vi "Teleop.vi"(10 "Match Info":T1={"Autonomous Elapsed Seconds"=0.0, "TeleOp Elapsed Seconds"=0.0, "Disabled Elapsed Seconds"=0.0, "Visited Autonomous"=FALSE, "Visited TeleOp"=FALSE, "Visited Disabled"=FALSE, "Autonomous Settings"={"Autonomous Style"=enum."Independent", "VI Refnum"=refnum}}, 11 "Call Context":T2) -> ()   [LabVIEW 2013]
doc: "This VI is called for each TeleOp packet received from the DS where the robot is not disabled. It is often used to read from the joysticks and update I/O or to update setpoints for timed control loops. It should complete and return within 20 milliseconds or it may miss DS packets."
uses:
  <vilib>/Rock Robotics/WPI/DriverStation/WPI_DriverStationDerivedRobotMode.ctl
  <vilib>/Rock Robotics/WPI/DriverStation/WPI_DriverStationMatch Info.ctl
  <vilib>/Rock Robotics/WPI/Relay/WPI_RelayValue.ctl
  <vilib>/Rock Robotics/WPI/DriverStation/DriverStationLCD/WPI_DriverStationLCDLCDLine.ctl
  <vilib>/Rock Robotics/WPI/Solenoid/WPI_SolenoidValue.ctl
  Robot Global Data.vi
  <vilib>/Rock Robotics/WPI/Solenoid/WPI_SolenoidSetEnum.vi
  <vilib>/Rock Robotics/WPI/Joystick/WPI_JoystickGetSetRefNum.vi
  <vilib>/Rock Robotics/WPI/Compressor/WPI_CompressorGetSetRefNum.vi
  <vilib>/Rock Robotics/WPI/RobotDrive/WPI_RobotDriveGetSetRefNum.vi
panel:
  out "Numeric 1":dbl(slide) scale=0.0..100.0
  out "Boolean 2":bool
  out "Boolean 1":bool
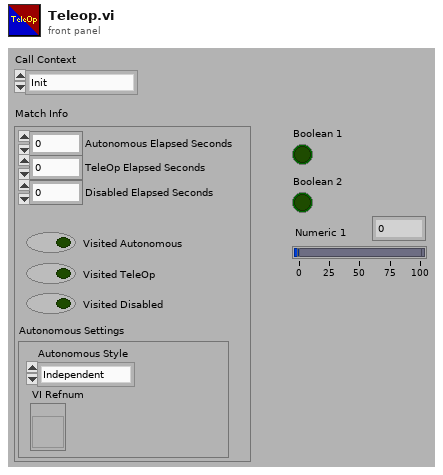
[diagram p1: front panel]
types:
  T1 = typedef "WPI_DriverStationMatch Info.ctl" = cluster{"Autonomous Elapsed Seconds":dbl, "TeleOp Elapsed Seconds":dbl, "Disabled Elapsed Seconds":dbl, "Visited Autonomous":bool, "Visited TeleOp":bool, "Visited Disabled":bool, "Autonomous Settings":cluster{"Autonomous Style":enum16{"Iterative", "Independent"}, "VI Refnum":refnum<vi>}}
  T2 = typedef "WPI_DriverStationDerivedRobotMode.ctl" = enum16{"Init", "Execute", "Stop"}
  T3 = typedef "WPI_JoystickDevRef.ctl" = cluster{"Device":T4}
  T4 = typedef "WPI_JoystickDeviceEnum.ctl" = enum16{"USB 1", "USB 2", "USB 3", "USB 4", "Kinect 1", "Kinect 2"}
  T5 = typedef "WPI_JoystickButtonState.ctl" = cluster{"Button 1":bool, "Button 2":bool, "Button 3":bool, "Button 4":bool, "Button 5":bool, "Button 6":bool, "Button 7":bool, "Button 8":bool, "Button 9":bool, "Button 10":bool, "Button 11":bool, "Button 12":bool}
  T6 = cluster{"axis 1 (x)":dbl, "axis 2 (y)":dbl, "axis 3 (throttle)":dbl, "axis 4":dbl, "axis 5":dbl, "axis 6":dbl}
  T7 = cluster{"Driver Station Digital Input (1-8)[0]":bool, "Driver Station Digital Input (1-8)[1]":bool, "Driver Station Digital Input (1-8)[2]":bool, "Driver Station Digital Input (1-8)[3]":bool, "Driver Station Digital Input (1-8)[4]":bool, "Driver Station Digital Input (1-8)[5]":bool, "Driver Station Digital Input (1-8)[6]":bool, "Driver Station Digital Input (1-8)[7]":bool, "Driver Station Digital Input (1-8)[8]":bool}
  T8 = typedef "WPI_CompressorDevRef.ctl" = cluster{"DevStatus":errorcluster, "DigitalInputDevRef":T9, "RelayDevRef":T12}
  T9 = typedef "WPI_DigitalInputDevRef.ctl" = cluster{"DevStatus":errorcluster, "DIO Channel":T10, "Digital Module":T11}
  T10 = typedef "FPGA_DIOChannel.ctl" = enum8{"DIO 1", "DIO 2", "DIO 3", "DIO 4", "DIO 5", "DIO 6", "DIO 7", "DIO 8", "DIO 9", "DIO 10", "DIO 11", "DIO 12", "DIO 13", "DIO 14", "Invalid"}
  T11 = typedef "FPGA_TypedefDigitalModule.ctl" = enum16{"Digital Module 1", "Digital Module 2"}
  T12 = typedef "WPI_RelayDevRef.ctl" = cluster{"DevStatus":errorcluster, "Relay Channel":T13, "Digital Module":T11, "Relay Direction":T14}
  T13 = typedef "FPGA_DIORelayChannel.ctl" = enum8{"Relay 1", "Relay 2", "Relay 3", "Relay 4", "Relay 5", "Relay 6", "Relay 7", "Relay 8", "Invalid"}
  T14 = typedef "WPI_RelayDirection.ctl" = enum16{"Both directions", "Forward only", "Reverse only"}
  T15 = typedef "WPI_SolenoidValue.ctl" = enum16{"Off", "On", "Forward", "Reverse"}
  T16 = typedef "WPI_DriverStationLCDLCDLine.ctl" = enum16{"Main - Line 1", "User - Line 2", "User - Line 3", "User - Line 4", "User - Line 5", "User - Line 6"}
  T17 = typedef "WPI_RelayValue.ctl" = enum16{"Off", "On", "Forward", "Reverse"}
  T18 = typedef "WPI_RobotDriveDevRef.ctl" = cluster{"DevStatus":errorcluster, "Motors[]":T19[], "Square Inputs":bool, "Max Output":dbl, "Isochronous":bool}
  T19 = typedef "WPI_MotorControlDeviceRef.ctl" = cluster{"DeviceStatus":errorcluster, "Type":enum16{"PWM", "CAN"}, "PWM":cluster{"Digital Module":T11, "PWM Channel":T20, "DeadBand":T21}, "CAN":cluster{"Device Number":u8, "Control Mode":T22, "Semaphore":T23, "Max Vout":dbl}, "Invert":bool, "TransformRef":T24, "InvTransformRef":T24}
  T20 = typedef "FPGA_DIOPWMChannel.ctl" = enum8{"PWM 1", "PWM 2", "PWM 3", "PWM 4", "PWM 5", "PWM 6", "PWM 7", "PWM 8", "PWM 9", "PWM 10", "Invalid"}
  T21 = typedef "WPI_PWMDeadband.ctl" = cluster{"Name":string, "maxPositivePwm":i32, "minPositivePwm":i32, "centerPwm":i32, "maxNegativePwm":i32, "minNegativePwm":i32, "angularRange":u16}
  T22 = typedef "WPI_CANJaguar_ControlMode.ctl" = enum8{"Percent VBus", "Current", "Speed", "Position", "Voltage"}
  T23 = typedef "Semaphore RefNum" = refnum<k1>
  T24 = typedef "WPI_PWMTransform_ConPane.ctl" = refnum<vi>
  T25 = typedef "WPI_SolenoidDevRef.ctl" = cluster{"DevStatus":errorcluster, "Solenoid Module":T26, "Forward Solenoid Channel":T27, "Reverse Solenoid Channel":T27}
  T26 = typedef "FPGA_TypedefSolenoidModule.ctl" = enum16{"Solenoid Module 1", "Solenoid Module 2"}
  T27 = typedef "WPI_SolenoidChannel.ctl" = enum8{"Solenoid 1", "Solenoid 2", "Solenoid 3", "Solenoid 4", "Solenoid 5", "Solenoid 6", "Solenoid 7", "Solenoid 8", "Invalid"}
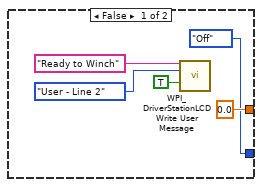
[diagram p2: hidden frame]
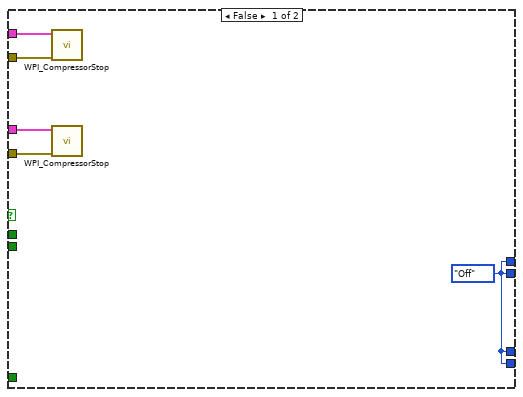
[diagram p3: hidden frame]
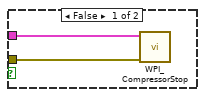
[diagram p4: hidden frame]
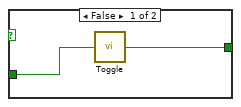
[diagram p7: hidden frame]
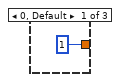
[diagram p8: hidden frame]
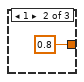
[diagram p9: hidden frame]
diagram:
  # "Read Joystick X and Y values and update motor values"
  n1 = call <vilib>:"WPI_DriverStationReport Robot Code State.vi"("TeleOp"=TRUE ("Autonomous")) -> ()  [unwired: 10 in, 1 out]
  n2 = global write "Robot Global Data.vi" "LED toggle rate (ms)"(u32 100 ("LED ms toggle rate")) -> ()
  n3 = call <vilib>:"SD Read Number.vi"("Name"="Slider 1" ("refnum name")) -> ("Numeric"=→"Numeric 1":dbl)  [unwired: 8 in, 2 out]
  n4 = Unbundle By Name("Match Info") -> ()  [unwired: 1 out]
  n5 = call <vilib>:"SD Read Boolean.vi"("Name"="Checkbox 1" ("refnum name")) -> ("Boolean"=→"Boolean 1":bool)  [unwired: 8 in, 2 out]
  n6 = call <vilib>:"SD Read Boolean.vi"("Name"="Checkbox 2" ("refnum name")) -> ("Boolean"=→"Boolean 2":bool)  [unwired: 8 in, 2 out]
  n7 = call <vilib>:"WPI_JoystickRefNum Registry Get.vi"("refnum name"="Left Joystick") -> ("JoystickDevRef"=w94:T3)  [unwired: 1 in, 9 out]
  n8 = call <vilib>:"WPI_JoystickRefNum Registry Get.vi"("refnum name"="Right Joystick") -> ("JoystickDevRef"=w76:T3)  [unwired: 1 in, 9 out]
  n9 = call <vilib>:"WPI_JoystickGet.vi"("JoystickDevRef"=w94) -> ("Buttons"=w74:T5, "Axes"=w89:T6)  [unwired: 1 in, 4 out]
  n10 = call <vilib>:"WPI_JoystickGet.vi"("JoystickDevRef"=w76) -> ("Buttons"=w73:T5, "Axes"=w72:T6)  [unwired: 1 in, 4 out]
  n11 = Unbundle By Name(w89) -> ("axis 2 (y)"=w63:dbl)
  n12 = Unbundle By Name(w74) -> ("Button 1"=w57:bool)
  n13 = Unbundle By Name(w72) -> ("axis 2 (y)"=w62:dbl)
  n14 = Unbundle By Name(w73) -> ("Button 1"=w52:bool)
  n15 = Cluster To Array(cluster=w89) -> (array=w88:dbl[])
  n16 = Cluster To Array(cluster=w74) -> (array=w91:bool[])
  n17 = call <vilib>:"WPI_DriverStationGet Digital Input.vi"() -> ("Driver Station Digital Input (1-8)"=w71:bool[])  [unwired: 11 in]
  n18 = Boolean To (0,1)(Boolean=w57) -> (0, 1=w55:i16)
  n19 = Boolean To (0,1)(Boolean=w52) -> (0, 1=w56:i16)
  n20 = Array To Cluster(array=w71) -> (cluster=w70:T7)
  n21 = call <vilib>:"WPI_CompressorRefNum Registry Get.vi"("refnum name"="Compressor") -> ("error out"=w50:errorcluster, "CompressorDevRef"=w49:T8)  [unwired: 9 in]
  n22 = call <vilib>:"SD Write Numeric Array.vi"("Numeric Array"=w88, "Name"="Joystick 1/Axes") -> ()  [unwired: 8 in, 2 out]
  n23 = Unbundle By Name(w70) -> ("Driver Station Digital Input (1-8)[0]"=w69:bool, "Driver Station Digital Input (1-8)[1]"=w33:bool, "Driver Station Digital Input (1-8)[2]"=w30:bool, "Driver Station Digital Input (1-8)[3]"=w29:bool, "Driver Station Digital Input (1-8)[4]"=w24:bool)
  n24 = call <vilib>:"SD Write Boolean Array.vi"("Boolean Array"=w91, "Name"="Joystick 1/Buttons") -> ()  [unwired: 8 in, 2 out]
  n25 = Add(x=w56, y=w55) -> (x+y=w54:i16)
  n26 = call <vilib>:"WPI_CompressorStart.vi"("error in (no error)"=w50, "CompressorDevRef"=w49) -> ("error out"=w25:errorcluster, "CompressorDevRef"=w26:T8)  [unwired: 8 in]
  n27 = call <vilib>:"WPI_CompressorRefNum Registry Get.vi"("refnum name"="Offboard Compressor") -> ("error out"=w27:errorcluster, "CompressorDevRef"=w28:T8)  [unwired: 9 in]
  n28 = case shown="True" w33 {
    tunnel: [w102 w115] -> w35
    tunnel: [w102 w114] -> w34
    tunnel: [w102 w111] -> w32
    tunnel: [w102 w110] -> w31
    tunnel: w30 -> [_ w109]
    tunnel: w29 -> [_ w108]
    tunnel: w28 -> [w101 w105]
    tunnel: w27 -> [w100 w104]
    tunnel: w26 -> [w99 w107]
    tunnel: w25 -> [w98 w106]
    tunnel: w24 -> [_ w103]
    frame False {
      w102 = WPI_SolenoidValue."Off" ("Value")
      n29 = call <vilib>:"WPI_CompressorStop.vi"("error in (no error)"=w98, "CompressorDevRef"=w99) -> ()  [unwired: 8 in, 2 out]
      n30 = call <vilib>:"WPI_CompressorStop.vi"("error in (no error)"=w100, "CompressorDevRef"=w101) -> ()  [unwired: 8 in, 2 out]
    }
    frame True {
      w112 = WPI_SolenoidValue."Reverse" ("Value")
      w113 = WPI_SolenoidValue."Forward" ("Value")
      n31 = call <vilib>:"WPI_CompressorStart.vi"("error in (no error)"=w106, "CompressorDevRef"=w107) -> ()  [unwired: 8 in, 2 out]
      n32 = case shown="True" w103 {
        tunnel: w105 -> [w117 w119]
        tunnel: w104 -> [w116 w118]
        frame False {
          n33 = call <vilib>:"WPI_CompressorStop.vi"("error in (no error)"=w116, "CompressorDevRef"=w117) -> ()  [unwired: 8 in, 2 out]
        }
        frame True {
          n34 = call <vilib>:"WPI_CompressorStart.vi"("error in (no error)"=w118, "CompressorDevRef"=w119) -> ()  [unwired: 8 in, 2 out]
        }
      }
      n35 = case shown="False" w109 {
        tunnel: w113 -> [_ w122]
        tunnel: [w120 w122] -> w111
        tunnel: w112 -> [_ w121]
        tunnel: [w120 w121] -> w110
        frame False {
          w120 = WPI_SolenoidValue."Off" ("Value")
        }
        frame True {
        }
      }
      n36 = case shown="False" w108 {
        tunnel: w113 -> [_ w125]
        tunnel: [w123 w125] -> w115
        tunnel: w112 -> [_ w124]
        tunnel: [w123 w124] -> w114
        frame False {
          w123 = WPI_SolenoidValue."Off" ("Value")
        }
        frame True {
        }
      }
    }
  }
  n37 = case shown="2" w54 {
    tunnel: [1 0.8 0.6] -> w53
    frame 0, Default {
    }
    frame 1 {
    }
    frame 2 {
    }
  }
  n38 = call <vilib>:"WPI_JoystickRefNum Registry Get.vi"("refnum name"="Gamepad") -> ("JoystickDevRef"=w67:T3)  [unwired: 1 in, 9 out]
  n39 = call <vilib>:"WPI_JoystickGet.vi"("JoystickDevRef"=w67) -> ("Buttons"=w66:T5, "Axes"=w65:T6)  [unwired: 1 in, 4 out]
  n40 = Unbundle By Name(w65) -> ("axis 2 (y)"=w59:dbl, "axis 5"=w58:dbl)  [unwired: 4 out]
  n41 = Unbundle By Name(w66) -> ("Button 1"=w47:bool, "Button 2"=w46:bool, "Button 3"=w6:bool, "Button 4"=w8:bool, "Button 5"=w12:bool, "Button 6"=w13:bool)
  n42 = case shown="False" w69 {
    tunnel: [w132 w135] -> w61
    tunnel: [w129 w134] -> w60
    tunnel: w63 -> [w133 _]
    tunnel: w62 -> [w131 _]
    tunnel: w59 -> [_ w135]
    tunnel: w58 -> [_ w134]
    tunnel: w53 -> [w130 _]
    frame False {
      n43 = Multiply(x=w133, y=w130) -> (x*y=w132:dbl)
      n44 = Multiply(x=w131, y=w130) -> (x*y=w129:dbl)
    }
    frame True {
    }
  }
  n45 = call "Toggle.vi"("Input"=w8) -> ("Output"=w7:bool)
  n46 = call "Toggle.vi"("Input"=w47) -> ("Output"=w36:bool)
  n47 = Select(t=1.0, s=w13, f=0.0) -> (s? t:f=w16:dbl)
  n48 = Select(t=-1.0, s=w12, f=0.0) -> (s? t:f=w15:dbl)
  n49 = case shown="True" w36 {
    tunnel: w46 -> [w137 _]
    tunnel: [w136 FALSE] -> w37
    frame False {
      n50 = call "Toggle.vi"("Input"=w137) -> ("Output"=w136:bool)
    }
    frame True {
    }
  }
  n51 = case shown="True" w7 {
    tunnel: w6 -> [_ w146]
    tunnel: [0.0 ("Output") w145] -> w5
    tunnel: [WPI_RelayValue."Off" ("RelayValue") WPI_RelayValue."Forward" ("RelayValue")] -> w1
    frame False {
      n52 = call <vilib>:"WPI_DriverStationLCDWrite User Message.vi"("line text"="Ready to Winch", "line"=WPI_DriverStationLCDLCDLine."User - Line 2", "clear line before write (T)"=TRUE) -> ()  [unwired: 12 in, 1 out]
    }
    frame True {
      n53 = Select(t=1.0, s=w146, f=0.0) -> (s? t:f=w145:dbl)
      n54 = call <vilib>:"WPI_DriverStationLCDWrite User Message.vi"("line text"="Winching...", "line"=WPI_DriverStationLCDLCDLine."User - Line 2", "clear line before write (T)"=TRUE) -> ()  [unwired: 12 in, 1 out]
    }
  }
  n55 = Add(x=w16, y=w15) -> (x+y=w14:dbl)
  n56 = call <vilib>:"WPI_RobotDriveRefNum Registry Get.vi"("refnum name"="Drive 4") -> ("RobotDriveDevRef"=w77:T18)  [unwired: 1 in, 9 out]
  n57 = call <vilib>:"WPI_RobotDriveRefNum Registry Get.vi"("refnum name"="Drive 2") -> ("RobotDriveDevRef"=w78:T18)  [unwired: 1 in, 9 out]
  n58 = call <vilib>:"WPI_MotorControlRefNum Registry Get.vi"("refnum name"="Roller") -> ("error out"=w23:errorcluster, "MotorControlDevRef"=w22:T19)  [unwired: 9 in]
  n59 = call <vilib>:"WPI_RobotDriveTankDrive.vi"("Right axis value"=w60, "Left axis value"=w61, "RobotDriveDevRef"=w78) -> ()  [unwired: 6 in, 3 out]
  n60 = call <vilib>:"WPI_MotorControlSetOutput.vi"("error in (no error)"=w23, "Output"=w14, "MotorControlDevRef"=w22) -> ()  [unwired: 6 in, 3 out]
  n61 = call <vilib>:"WPI_RobotDriveTankDrive.vi"("Right axis value"=w60, "Left axis value"=w61, "RobotDriveDevRef"=w77) -> ("Motor Values"=w64:dbl[])  [unwired: 6 in, 2 out]
  n62 = call <vilib>:"SD Write Numeric Array.vi"("Numeric Array"=w64, "Name"="RobotDrive Motors") -> ()  [unwired: 8 in, 2 out]
  n63 = Select(t=w32, s=w36, f=w31) -> (s? t:f=w39:T15)
  n64 = Select(t=w35, s=w37, f=w34) -> (s? t:f=w38:T15)
  n65 = call <vilib>:"WPI_SolenoidRefNum Registry Get.vi"("refnum name"="Chomp") -> ("error out"=w41:errorcluster, "SolenoidDevRef"=w40:T25)  [unwired: 9 in]
  n66 = call-poly <vilib>:"WPI_SolenoidSet.vi"("error in (no error)"=w41, "Value"=w38, "SolenoidDevRef"=w40) -> ()  [unwired: 7 in, 2 out]
  n67 = call <vilib>:"WPI_MotorControlRefNum Registry Get.vi"("refnum name"="Winch") -> ("error out"=w9:errorcluster, "MotorControlDevRef"=w10:T19)  [unwired: 9 in]
  n68 = call <vilib>:"WPI_RelayRefNum Registry Get.vi"("refnum name"="Winch Clutch") -> ("error out"=w3:errorcluster, "RelayDevRef"=w2:T12)  [unwired: 9 in]
  n69 = call <vilib>:"WPI_SolenoidRefNum Registry Get.vi"("refnum name"="Claw") -> ("error out"=w43:errorcluster, "SolenoidDevRef"=w42:T25)  [unwired: 9 in]
  n70 = call-poly <vilib>:"WPI_SolenoidSet.vi"("error in (no error)"=w43, "Value"=w39, "SolenoidDevRef"=w42) -> ()  [unwired: 7 in, 2 out]
  n71 = call <vilib>:"WPI_MotorControlSetOutput.vi"("error in (no error)"=w9, "Output"=w5, "MotorControlDevRef"=w10) -> ()  [unwired: 6 in, 3 out]
  n72 = call <vilib>:"WPI_RelaySet.vi"("error in (no error)"=w3, "RelayValue"=w1, "RelayDevRef"=w2) -> ()  [unwired: 7 in, 2 out]
